vi "LCD Controller.vi"() -> ()   [LabVIEW 2012]
uses:
  Type/_RT Command.ctl
  Type/_RT Serial Command.ctl
panel:
  in  "Send":bool
  in  "Message to  Display":string="Welcome"
  out "Telegram":string
  in  "Contrast Value":u8=128
  in  "Command":T1(ring)
  # "For the RS232-2 serial chanel supported through FPGA using pins:\nPort 6.1 for RXD and 6.2 for TXD"
  # "(Maximum of 40 characters)"
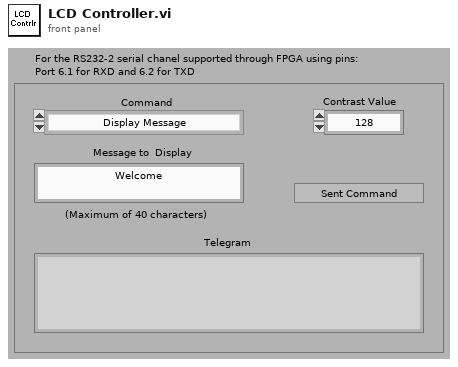
[diagram p1: front panel]
types:
  T1 = enum16{"Display Message", "Clear Display", "Set Contrast", "Set Contrast and Save", "Backlight On", "Backlight Off"}
  T2 = typedef "_RT Serial Command.ctl" = cluster{"Port Type":u16, "baud rate (9600)":u32, "data bits (8)":u16, "stop bits (1)":u16, "parity (0:none)":u16, "DoRead":bool, "Command":string}
  T3 = typedef "_RT Command.ctl" = enum16{"Start", "Stop", "Runtime Update", "Get Data", "Get Info", "Get Status", "Get Param", "Get Config", "Get Table", "Read ADC", "Set Oscillator", "Update Config", "Update Table", "Set All Pol", "Set Pol and DC", "Set Max Mass", "Toggle RP", "Toggle EL", "Set PIC", "Initialize Turbo", "Send Turbo Comm", "Close Turbo", "P1", "P2", "P3", "Send Serial", "Set LC Out", "Get LC In", "Read VAC", "Test Table", "Toggle Power", "Get Startup", "Set Startup", "Get ADC Table", "Set ADC Table", "Get Brief Status", "Get Detail Status", "Auxiliary Update", "Set CC Logics", "Set CC Input Logics", "Ignore Error"}
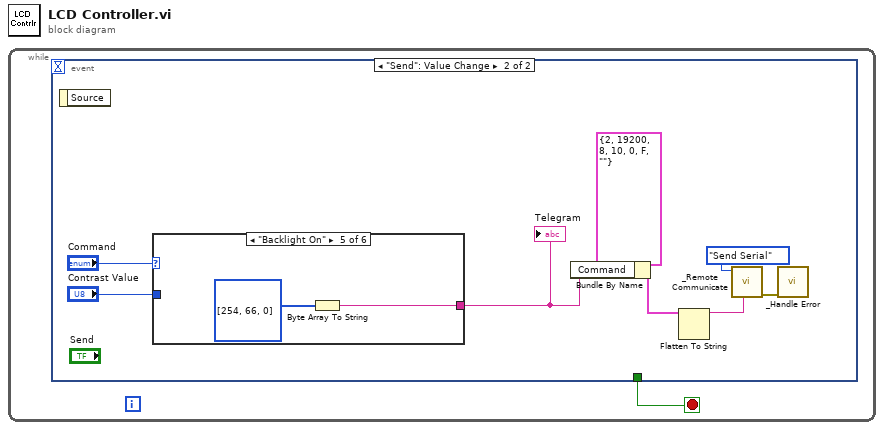
[diagram p0: block diagram]
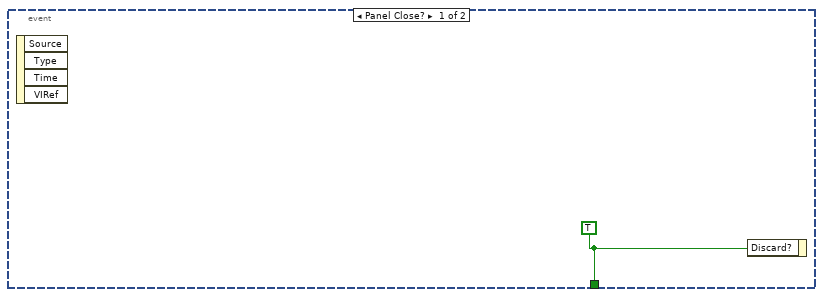
[diagram p2: hidden frame]
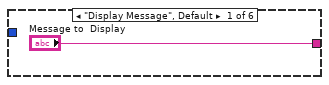
[diagram p3: hidden frame]
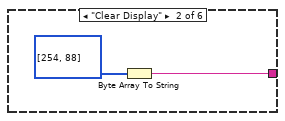
[diagram p4: hidden frame]
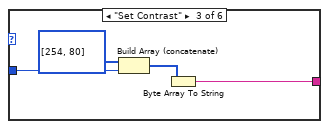
[diagram p5: hidden frame]
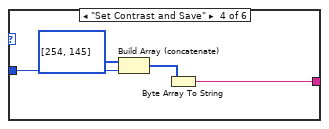
[diagram p6: hidden frame]
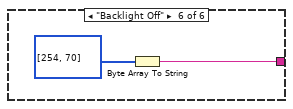
[diagram p7: hidden frame]
diagram:
  n1 = while {
    stop <- w1 stop-if-true
    n2 = event shown="[1] \"Send\": Value Change" {
      selector: _ -> [_ _]
      dyn-events: _ -> [_ _]
      timeout: _ -> [_ _]
      tunnel: [w2 _] -> w1
      event Panel Close? {
        w2 = TRUE
        n3 = event-data() -> ()  [unwired: 5 out]
        n4 = event-data("Discard?"=w2) -> ()  [unwired: 1 in, 1 out]
      }
      event "Send": Value Change {
        n5 = event-data() -> ()  [unwired: 2 out]
        n6 = case shown="\"Backlight On\"" "Command" {
          tunnel: "Contrast Value" -> [_ _ w15 w19 _ _]
          tunnel: ["Message to  Display" w12 w17 w21 w23 w25] -> w3
          frame "Display Message", Default {
          }
          frame "Clear Display" {
            n7 = Byte Array To String(unsigned byte array=u8[] [254, 88]) -> (string=w12:string)
          }
          frame "Set Contrast" {
            n8 = Build Array (concatenate)(u8[] [254, 80], w15) -> (w14:u8[])
            n9 = Byte Array To String(unsigned byte array=w14) -> (string=w17:string)
          }
          frame "Set Contrast and Save" {
            n10 = Build Array (concatenate)(u8[] [254, 145], w19) -> (w18:u8[])
            n11 = Byte Array To String(unsigned byte array=w18) -> (string=w21:string)
          }
          frame "Backlight On" {
            n12 = Byte Array To String(unsigned byte array=u8[] [254, 66, 0]) -> (string=w23:string)
          }
          frame "Backlight Off" {
            n13 = Byte Array To String(unsigned byte array=u8[] [254, 70]) -> (string=w25:string)
          }
        }
        "Telegram" <- w3
        n14 = Bundle By Name(cluster=T2 {"Port Type"=2, "baud rate (9600)"=19200, "data bits (8)"=8, "stop bits (1)"=10, "parity (0:none)"=0, "DoRead"=FALSE, "Command"=""} ("Serial Command"), "Command"=w3) -> (w5:T2)
        n15 = Flatten To String(anything=w5) -> (data string=w10:string)  [unwired: 1 in, 4 out]
        n16 = call "_Remote Communicate.vi"("String"=w10, "Command"=_RT_Command."Send Serial") -> ("error out"=w8:errorcluster)  [unwired: 4 in, 3 out]
        n17 = call "_Handle Error.vi"("error in (no error)"=w8) -> ()  [unwired: 2 in, 5 out]
      }
    }
  }
